vi "3D Rotation.vi"(7 "Angles":sgl[](array[numeric])) -> (8 "axis":cluster{"X":sgl, "Y":sgl, "Z":sgl}, 10 "angle":dbl)   [LabVIEW 2023]
uses:
  <vilib>/Analysis/coordinate.llb/Euler Rotation Order.ctl
  <vilib>/Analysis/NI_AALPro.lvlib
  <vilib>/Analysis/NI_AALBase.lvlib
  <vilib>/Analysis/baseanly.llb/Real Dot Product.vi
  <vilib>/Analysis/coordinate.llb/3D Cartesian Coordinate Rotation (Euler) (Scalar).vi
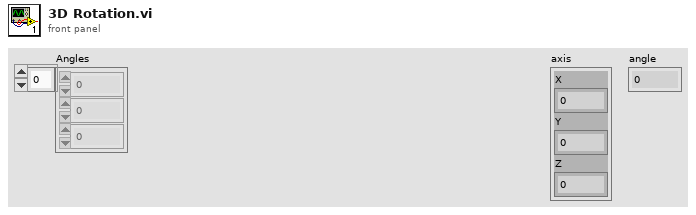
[diagram p1: front panel]
types:
  T1 = typedef "NI_AALPro.lvlib/Euler Rotation Order.ctl" = u16
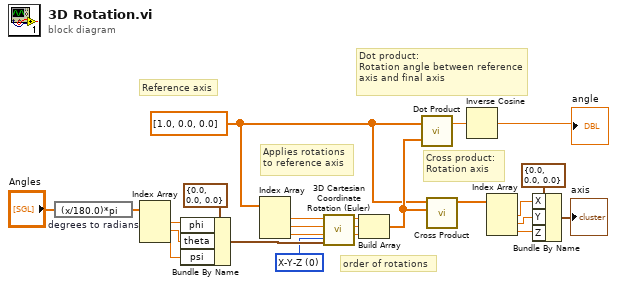
[diagram p0: block diagram]
diagram:
  w1 = sgl[] [1.0, 0.0, 0.0]
  w19 = T1 0 items=["X-Y-Z", "X-Z-Y", "Y-X-Z", "Y-Z-X", "Z-X-Y", "Z-Y-X", "X-Y-X", "X-Z-X", "Y-X-Y", "Y-Z-Y", "Z-X-Z", "Z-Y-Z"] ("rotation order")
  # "order of rotations"
  # "Cross product:\nRotation axis"
  # "Applies rotations\nto reference axis"
  # "Reference axis"
  # "Dot product:\nRotation angle between reference axis and final axis"
  n1 = expression code="(x/180.0)*pi" "degrees to radians"("Angles") -> (w13:sgl[])
  n2 = Index Array(array=w13) -> (element #1=w21:sgl, element #2=w22:sgl, element #3=w23:sgl)  [unwired: 3 in]
  n3 = Bundle By Name(cluster=cluster{"phi":dbl, "theta":dbl, "psi":dbl} {"phi"=0.0, "theta"=0.0, "psi"=0.0} ("Euler Angles"), "phi"=w21, "theta"=w22, "psi"=w23) -> (w24:cluster{"phi":dbl, "theta":dbl, "psi":dbl})
  n4 = Index Array(array=w1) -> (element #1=w9:sgl, element #2=w7:sgl, element #3=w8:sgl)  [unwired: 3 in]
  n5 = call-poly <vilib>:"3D Cartesian Coordinate Rotation (Euler).vi"("rotation order"=w19, "Euler Angles"=w24, "z"=w8, "y"=w7, "x"=w9) -> ("z out"=w12:dbl, "y out"=w11:dbl, "x out"=w10:dbl)  [unwired: 3 in, 1 out]
  n6 = Build Array(w10, w11, w12) -> (w5:dbl[])
  n7 = call-poly <vilib>:"Dot Product.vi"("Y Vector"=w5, "X Vector"=w1) -> ("X * Y"=w18:dbl)  [unwired: 1 out]
  n8 = call <vilib>:"Cross Product.vi"("B Vector"=w5, "A Vector"=w1) -> ("Cross Product"=w6:dbl[])  [unwired: 8 in, 1 out]
  n9 = Inverse Cosine(1:w18) -> (0:→"angle":dbl)
  n10 = Index Array(array=w6) -> (element #1=w16:dbl, element #2=w15:dbl, element #3=w14:dbl)  [unwired: 3 in]
  n11 = Bundle By Name(cluster=cluster{"X":sgl, "Y":sgl, "Z":sgl} {"X"=0.0, "Y"=0.0, "Z"=0.0} ("Axis"), "X"=w16, "Y"=w15, "Z"=w14) -> (→"axis":cluster{"X":sgl, "Y":sgl, "Z":sgl})
